vi "spilib_close.vi"(8 "error in (no error)":errorcluster, 11 "handle":i32) -> (0 "error out":errorcluster)   [LabVIEW 2017]
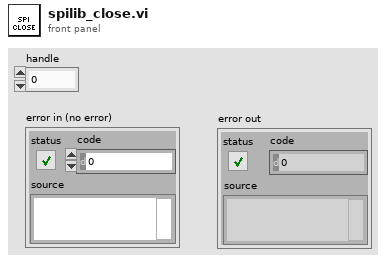
[diagram p1: front panel]
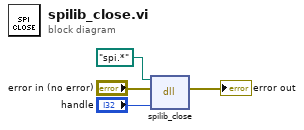
[diagram p0: block diagram]
diagram:
  n1 = dll-call lib="?" fn="spilib_close"(path in=path "spi.*", error in="error in (no error)", "handle"="handle") -> (error out=→"error out":errorcluster)  [unwired: 3 in, 1 out]
